vi "TestLQR.vi"() -> ()   [LabVIEW 2016]
uses:
  <vilib>/addons/control/pid/NI_PID_pid.lvlib
  <vilib>/Simulation/Implementation/XNodeFramework/SimXNode/SimX.xnode
  <vilib>/addons/control/pid/pid.llb/PID (DBL).vi
  <vilib>/rvi/Analysis/host/Private/Convert PID Gains (PID).vi
  <vilib>/Simulation/DiscreteLinear/Implementation/NILVSim Discrete Transfer Function Direct.llb/SIM Discrete Transfer Function Diagram (SISO).vi
  <vilib>/Simulation/Shared/_Datatypes/SIM SISO Transfer Function.ctl
panel:
  out "homemade pid":dbl
  in  "output range":cluster{"output high":dbl, "output low":dbl}={"output high"=100.0, "output low"=-100.0} {"output low" format="%.2f"; "output high" format="%.2f"}
  in  "reinitialize? (F)":bool
  in  "Loops":i32=4
  in  "initialize":bool
  out "output transfer func":dbl
  out "dt out (s)":dbl format="%.3f"
  in  "PID gains":T1={"proportional gain (Kc)"=1.0, "integral time (Ti, min)"=0.01, "derivative time (Td, min)"=0.0} {"derivative time (Td, min)" format="%.3f"; "integral time (Ti, min)" format="%.3f"; "proportional gain (Kc)" format="%.3f"}
  out "Output":dbl
  in  "Error":dbl
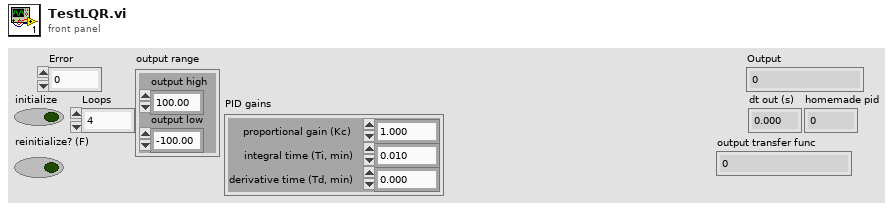
[diagram p1: front panel]
types:
  T1 = cluster{"proportional gain (Kc)":dbl, "integral time (Ti, min)":dbl, "derivative time (Td, min)":dbl}
  T2 = typedef "SIM SISO Transfer Function.ctl" = cluster{"Numerator":dbl[], "Denominator":dbl[]}
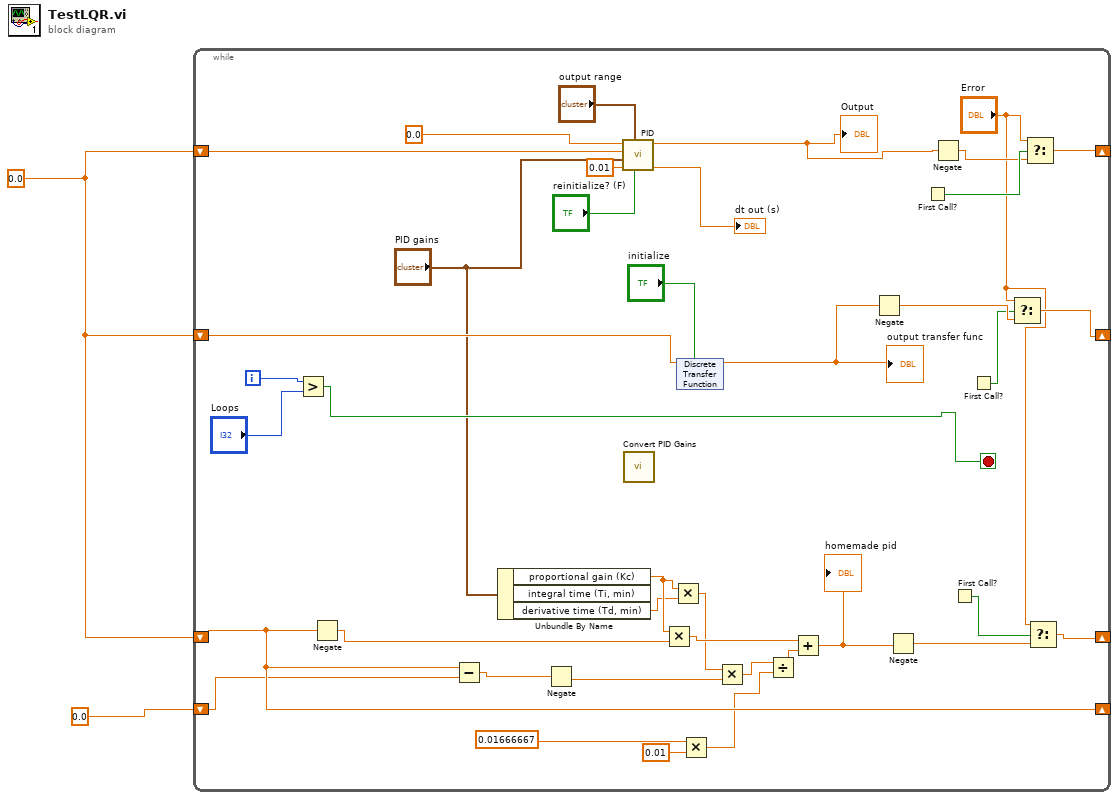
[diagram p0: block diagram]
diagram:
  w1 = 0.0 ("Error")
  n1 = while {
    shift-right: [w12] -> _
    shift-left: w1 -> [w37]
    shift-right: [w9] -> _
    shift-left: w1 -> [w34]
    shift-right: [w25] -> _
    shift-left: 0.0 ("Error") -> [w24]
    shift-right: [w6] -> _
    shift-left: w1 -> [w25]
    i -> [w39]
    stop <- w35 stop-if-true
    n2 = Greater?(x=w39, y="Loops") -> (0:w35:bool)
    n3 = Negate(x=w25) -> (-x=w27:dbl)
    n4 = Subtract(x=w25, y=w24) -> (x-y=w23:dbl)
    n5 = Unbundle By Name("PID gains") -> ("proportional gain (Kc)"=w22:dbl, "derivative time (Td, min)"=w21:dbl)  [unwired: 1 out]
    n6 = Negate(x=w23) -> (-x=w19:dbl)
    n7 = call-poly <vilib>:"PID.vi"("reinitialize? (F)"="reinitialize? (F)", "output range"="output range", "dt (s)"=0.01, "PID gains"="PID gains", "process variable"=w37, "setpoint"=0.0) -> ("dt out (s)"=→"dt out (s)":dbl, "output"=w30:dbl)  [unwired: 4 in]
    "Output" <- w30
    n8 = call-poly <vilib>:"Convert PID Gains.vi"() -> ()  [unwired: 14 in, 2 out]
    n9 = Multiply(x=w22, y=w27) -> (x*y=w26:dbl)
    n10 = Multiply(x=w22, y=w21) -> (x*y=w20:dbl)
    n11 = xnode "Discrete Transfer Function"("input u(k)"=w34, "initialize"="initialize") -> ("output y(k)"=w29:dbl)  [unwired: 1 in, 1 out]
    "output transfer func" <- w29
    n12 = Multiply(x=0.01666667, y=0.01) -> (x*y=w15:dbl)
    n13 = Multiply(x=w20, y=w19) -> (x*y=w17:dbl)
    n14 = Divide(x=w17, y=w15) -> (x/y=w18:dbl)
    n15 = Add(x=w26, y=w18) -> (x+y=w16:dbl)
    "homemade pid" <- w16
    n16 = Negate(x=w29) -> (-x=w8:dbl)
    n17 = Negate(x=w16) -> (-x=w4:dbl)
    n18 = First Call?() -> (First Call?: T/F=w11:bool)
    n19 = Negate(x=w30) -> (-x=w10:dbl)
    n20 = First Call?() -> (First Call?: T/F=w3:bool)
    n21 = First Call?() -> (First Call?: T/F=w7:bool)
    n22 = Select(t="Error", s=w7, f=w8) -> (s? t:f=w9:dbl)
    n23 = Select(t="Error", s=w11, f=w10) -> (s? t:f=w12:dbl)
    n24 = Select(t="Error", s=w3, f=w4) -> (s? t:f=w6:dbl)
  }
